vi "REC_Query NUM.vi"(0 "System no.":i32=1 min=1 max=4 step=1, 2 "RecorderIDs to query":string[](array[string]), 5 "error in":errorcluster) -> (14 "Number of recorded data points":i32[](array[numeric]), 19 "error out":errorcluster)   [LabVIEW 2020]
doc: "REC? NUM (Get Number of Recorded Data Points)\n\nDescription \nQueries the number of recorded data points for the specified data recorder or for all data \nrecorders in the controller.\nFor the queried data recorder, the returned number of data points applies to each of its data \nrecorder traces that contains recorded data.\n\nFormat\nREC? NUM[ <RecorderID>]\n\nArguments\nREC? NUM without arguments queries all data recorders of the controller. \n<RecorderID>\nData recorder to be queried; to be specified as alias (p. 94) \nThe available data recorders can be queried with USG? SYS (p. 80). \nPossible values: REC_1 to RECn, where n = number of data recorders in the controller\nResponse\n{<RecorderID> = <DataPoints> LF}\n- <DataPoints>: Number = 0; number of recorded data points\n\nExample\n>>rec? num\n<<REC_1=1562\n<<REC_2=0\n>>rec? num rec_1\n<<REC_1=1562\n>>rec? num rec_2\n<<REC_2=0\n\nNotes\nNote that the data in all traces of a data recorder will be deleted if the configuration of the data \nrecorder is changed. The configuration can be changed with REC TRG (p. 40), REC TRACE (p. 38) \nor REC RATE (p. 35), as well as via configuration parameters (p. 119). \nIf no trace of the data recorder contains data, REC? NUM responds with the value 0, and the \nquery of the data points with REC? DAT (p. 43) will fail for this data recorder.\nFor further details, see \"Data Recorder - GCS 3.0\" (p. 107). \n\nUser command level\nUSR"
panel:
  # "REC? NUM (Get Number of Recorded Data Points)\n\nQueries the number of recorded data points for the specified data recorder or for all data recorders in the controller.\nFor the queried data recorder, the returned number of data points applies to each of its data recorder traces that contains recorded data."
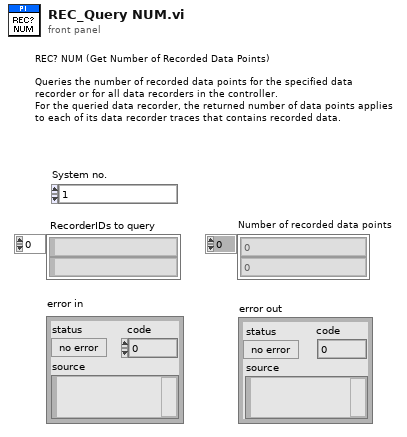
[diagram p1: front panel]
types:
  T1 = typedef "Syntax.ctl" = enum16{"GCS 1.0", "GCS 2.0", "GCS 3.0"}
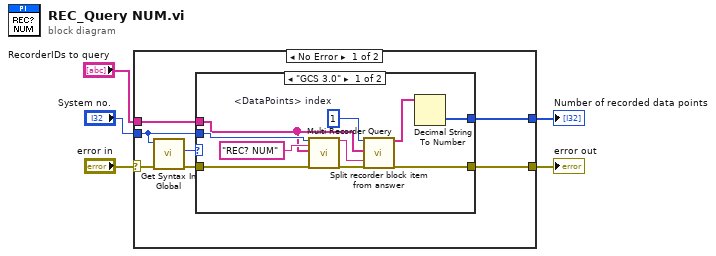
[diagram p0: block diagram]
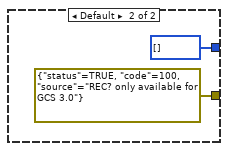
[diagram p2: hidden frame]
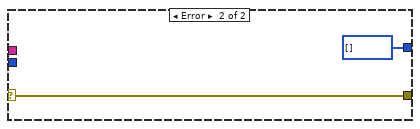
[diagram p3: hidden frame]
diagram:
  n1 = case shown="No Error" "error in" {
    selector: "error in" -> [w12 w26]
    tunnel: [w9 w26] -> w4
    tunnel: "RecorderIDs to query" -> [w7 _]
    tunnel: "System no." -> [w6 _]
    tunnel: [w8 i32[] [] ("Number of recorded data points")] -> w1
    frame No Error {
      n2 = call "Get Syntax In Global.vi"("error in"=w12, "System no."=w6) -> ("error out"=w10:errorcluster, "Syntax"=w11:T1)  [unwired: 8 in]
      n3 = case shown="\"GCS 3.0\"" w11 {
        tunnel: w10 -> [w20 _]
        tunnel: [w13 errorcluster {"status"=TRUE, "code"=100, "source"="REC? only available for GCS 3.0"} ("error out")] -> w9
        tunnel: [w17 i32[] [] ("Number of recorded data points")] -> w8
        tunnel: w7 -> [w16 _]
        tunnel: w6 -> [w22 _]
        frame "GCS 3.0" {
          w19 = 1  # <DataPoints> index
          n4 = call "Multi Recorder Query.vi"("System no."=w22, "Recorder Command"="REC? NUM" ("format string"), "RecorderIDs to query"=w16, "error in"=w20) -> ("Answer"=w15:string, "error out"=w14:errorcluster)  [unwired: 14 in]
          n5 = call "Split recorder block item from answer.vi"("Slice block item"=w19, "RecorderIDs to query"=w16, "Input string"=w15, "error in"=w14) -> ("Sliced text segments"=w18:string[], "error out"=w13:errorcluster)  [unwired: 14 in]
          n6 = Decimal String To Number(string=w18) -> (number=w17:i32[])  [unwired: 2 in, 1 out]
        }
        frame Default {
        }
      }
    }
    frame Error {
    }
  }
  "error out" <- w4
  "Number of recorded data points" <- w1
